vi "GetMaximumCurrent.vi"(11 "Properties":T1[](array[typedef])) -> (3 "Maximum Current (%FLA)":dbl=110.0)   [LabVIEW 2017, in "McsaAnalysisLowRate.lvlib"]
uses:
  <vilib>/addons/InsightCM/Devices/Shared/Mcsa/McsaAnalysisLowRate/McsaAnalysisLowRate.lvlib
  <vilib>/addons/InsightCM/MessageBus/Base/controls/KeyValuePair.ctl
  <vilib>/addons/InsightCM/Utilities/PropertyHelpers/PropertyHelpers.lvlib
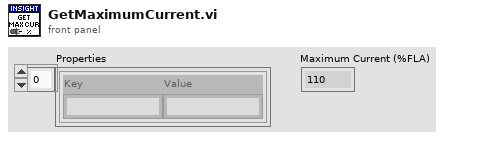
[diagram p1: front panel]
types:
  T1 = typedef "KeyValuePair.ctl" = cluster{"Key":string, "Value":string}
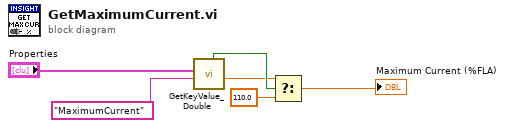
[diagram p0: block diagram]
diagram:
  n1 = call <vilib>:"GetKeyValue_Double.vi"("key"="MaximumCurrent", "key value pairs"="Properties") -> ("value"=w2:dbl, "found"=w5:bool)  [unwired: 7 in, 1 out]
  n2 = Select(t=w2, s=w5, f=110.0) -> (s? t:f=→"Maximum Current (%FLA)":dbl)
